vi "TL calculate power used.vi"(3 "Power in":dbl=5.0 format="%#_13g", 4 "Loop Time":u32, 5 "Speed":dbl=5.0 format="%#_13g") -> (0 "Power out":dbl, 2 "Speed out":dbl format="%#_13g")   [LabVIEW 2014]
doc: "This VI calculate the incremental power used during each simulation loop and adds it to create a total power used since the routine began. If the power level reaches 0 the speed will be set to zero."
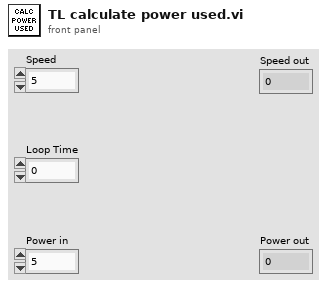
[diagram p1: front panel]
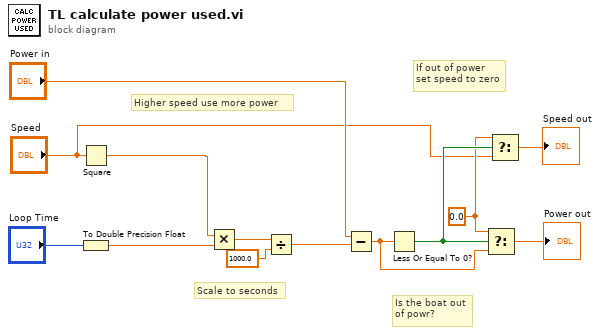
[diagram p0: block diagram]
diagram:
  w4 = 0.0
  # "Is the boat out\nof powr?"
  # "If out of power\nset speed to zero"
  # "Scale to seconds"
  # "Higher speed use more power"
  n1 = Square(x="Speed") -> (x^2=w3:dbl)
  n2 = To Double Precision Float(number="Loop Time") -> (double precision float=w10:dbl)
  n3 = Multiply(x=w3, y=w10) -> (x*y=w13:dbl)
  n4 = Divide(x=w13, y=1000.0) -> (x/y=w9:dbl)
  n5 = Subtract(x="Power in", y=w9) -> (x-y=w7:dbl)
  n6 = Less Or Equal To 0?(x=w7) -> (x <= 0?=w5:bool)
  n7 = Select(t=w4, s=w5, f=w7) -> (s? t:f=→"Power out":dbl)
  n8 = Select(t=w4, s=w5, f="Speed") -> (s? t:f=→"Speed out":dbl)
